vi "Start measurement.vi"(10 "Actual measurement":T2={"Start"=80.0, "Start Caption"="Start [T]", "End"=0.0, "End Caption"="End [T]", "Sweep"=0.0, "Sweep caption"="Rate [mT/s]", "Constant"=0.0, "Constant caption"="Freq [GHz]", "Mod_F [kHz]"=0.0, "Mod_A [G]"=0.001, "Tau [ms]"=0.0, "Angle [°]"=0.0, "Tmp [K]"=50.0, "Wait [min]"=0.0, "Carousel"=-1, "Comment"="", "Auto-mod"=TRUE, "Execute"=FALSE} {"Carousel" items=["0", "1", "2", "3", "4", "5", "6"]; "Angle [°]" min=0.0 max=350.0; "Tau [ms]" min=0.0 max=100.0; "Wait [min]" min=0.0 max=350.0; "Tmp [K]" min=0.0 max=3000.0; "Mod_A [G]" min=0.1 max=150.0; "Mod_F [kHz]" min=0.1 max=150.0}, 11 "Referencies in":T1) -> (0 "error out":errorcluster)   [LabVIEW 2024]
uses:
  Datatypes/script polymorh line.ctl
  Subsystem modules/Messenger service/Data types/Messenger referencies.ctl
  Subsystem modules/Magnet module/ctl/SetField data.ctl
  Subsystem modules/Magnet module/ctl/Magnet mode public.ctl
  Subsystem modules/Magnet module/ctl/MSG to magnet.ctl
  Subsystem modules/Magnet module/ctl/Magnet Orders.ctl
  Subsystem modules/Lock-in module/ctl/MFLI_parameter and value.ctl
  Subsystem modules/Lock-in module/ctl/MFLI_node.ctl
  Subsystem modules/Lock-in module/ctl/MFLI_message for module.ctl
  Subsystem modules/Lock-in module/ctl/MFLI_command enum.ctl
  Subsystem modules/Sample rotator/ctl/MSG to Rotator.ctl
  Subsystem modules/Sample rotator/ctl/Rotator commands.ctl
  Subsystem modules/Magnet module/Magnet module.lvlib
  Subsystem modules/Lock-in module/Lock-in module.lvlib
  Subsystem modules/Sample rotator/SampleRotator.lvlib
  Subsystem modules/Messenger service/MessengerLib.lvlib
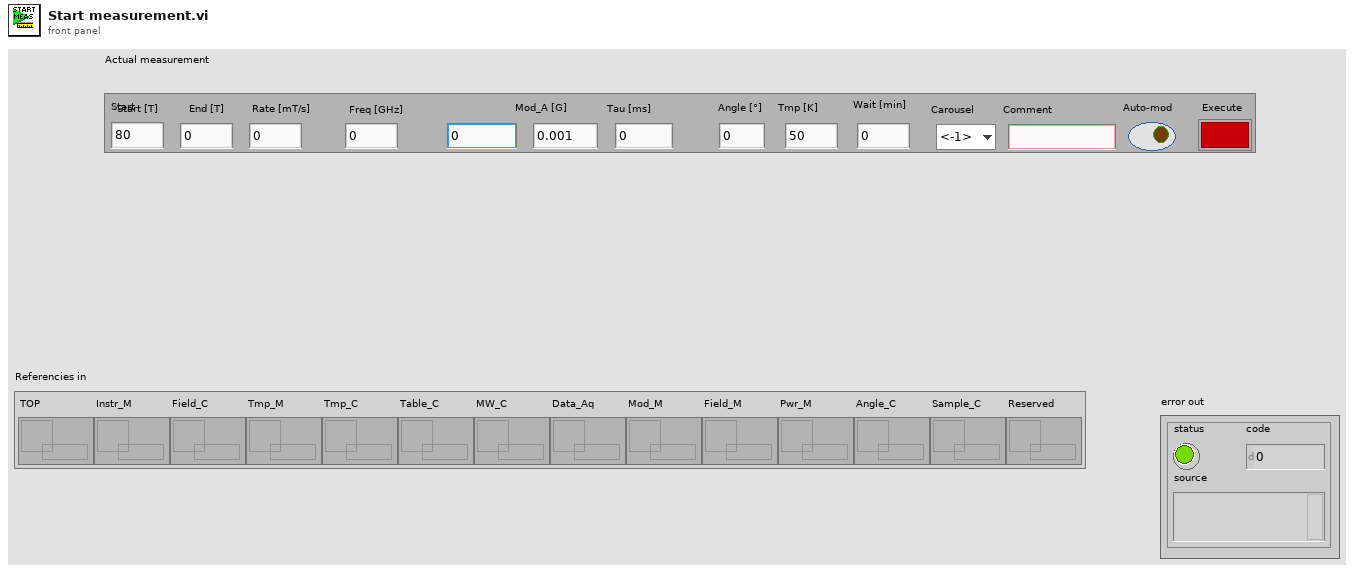
[diagram p1: front panel]
types:
  T1 = typedef "MessengerLib.lvlib/Messenger referencies.ctl" = cluster{"TOP":refnum<queue>, "Instr_M":refnum<queue>, "Field_C":refnum<queue>, "Tmp_M":refnum<queue>, "Tmp_C":refnum<queue>, "Table_C":refnum<queue>, "MW_C":refnum<queue>, "Data_Aq":refnum<queue>, "Mod_M":refnum<queue>, "Field_M":refnum<queue>, "Pwr_M":refnum<queue>, "Angle_C":refnum<queue>, "Sample_C":refnum<queue>, "Reserved":refnum<queue>}
  T2 = typedef "script polymorh line.ctl" = cluster{"Start":dbl, "Start Caption":string, "End":dbl, "End Caption":string, "Sweep":dbl, "Sweep caption":string, "Constant":dbl, "Constant caption":string, "Mod_F [kHz]":dbl, "Mod_A [G]":dbl, "Tau [ms]":dbl, "Angle [°]":dbl, "Tmp [K]":dbl, "Wait [min]":dbl, "Carousel":i8, "Comment":string, "Auto-mod":bool, "Execute":bool}
  T3 = typedef "Magnet module.lvlib/MSG to magnet.ctl" = cluster{"Order":T4, "Data":variant}
  T4 = typedef "Magnet module.lvlib/Magnet Orders.ctl" = enum16{"Ignore", "Connect", "Update", "Switch mode", "Set field", "Stop ramping", "Equalize output", "Zero output", "Flip polarity", "Blackout", "Set timer", "Eval temperatures", "Disconnect"}
  T5 = typedef "Lock-in module.lvlib/MFLI_message for module.ctl" = cluster{"Command":T6, "Data":variant}
  T6 = typedef "Lock-in module.lvlib/MFLI_command enum.ctl" = enum16{"Initialize", "Update", "Set parameters", "Set module", "Set individual parameters", "Get point", "Get array", "Disconnect", "End", "Ignore"}
  T7 = typedef "Lock-in module.lvlib/MFLI_parameter and value.ctl" = cluster{"parameter":T8, "value":dbl}
  T8 = typedef "Lock-in module.lvlib/MFLI_node.ctl" = enum16{"None", "filter_order [-]", "filter_constant [ms]", "in_diff", "in_autorange", "in_imp50", "in_AC", "osc_freq [kHz]", "out_ampl [V]", "out_autorange", "out_imp50", "enable output", "enamble ampl", "scope_enable", "scope_rate", "scope_len", "scope_trigEn", "AuxOut_amplify", "Phase_deg", "AuxOut_select"}
  T9 = typedef "Magnet module.lvlib/Magnet mode public.ctl" = enum16{"Persistant", "Ramping"}
  T10 = typedef "Magnet module.lvlib/SetField data.ctl" = cluster{"Field [T]":dbl, "Ramp [T/s]":dbl, "Custom Ramp?":bool, "Mode":T9}
  T11 = typedef "SampleRotator.lvlib/MSG to Rotator.ctl" = cluster{"Command":T12, "Data":variant}
  T12 = typedef "SampleRotator.lvlib/Rotator commands.ctl" = enum16{"Ignore", "Initialize", "Update", "Set parameters", "Stop movement", "Set position", "Disconnect", "End"}
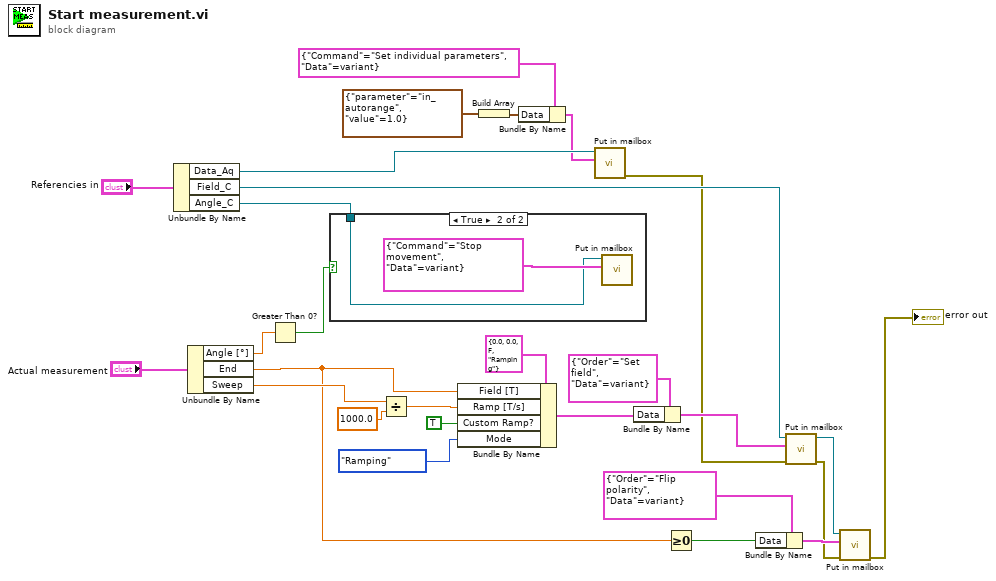
[diagram p0: block diagram]
diagram:
  n1 = Unbundle By Name("Referencies in") -> ("Data_Aq"=w14:refnum<queue>, "Field_C"=w7:refnum<queue>, "Angle_C"=w2:refnum<queue>)
  n2 = Unbundle By Name("Actual measurement") -> ("Angle [°]"=w3:dbl, "End"=w26:dbl, "Sweep"=w27:dbl)
  n3 = Greater Than 0?(x=w3) -> (x > 0?=w1:bool)
  n4 = case shown="True" w1 {
    tunnel: w2 -> [_ w29]
    frame False {
    }
    frame True {
      n5 = call "Put in mailbox.vi"("Message"=T11 {"Command"=enum."Stop movement", "Data"=variant} ("MSG to rotator"), "Queue in"=w29) -> ()  [unwired: 7 in, 3 out]
    }
  }
  n6 = Divide(x=w27, y=1000.0) -> (x/y=w23:dbl)
  n7 = Bundle By Name(cluster=T10 {"Field [T]"=0.0, "Ramp [T/s]"=0.0, "Custom Ramp?"=FALSE, "Mode"=enum."Ramping"} ("Set Field"), "Field [T]"=w26, "Ramp [T/s]"=w23, "Custom Ramp?"=TRUE, "Mode"=Magnet_mode_public."Ramping") -> (w22:T10)
  n8 = Build Array(T7 {"parameter"=enum."in_autorange", "value"=1.0} ("Parameter to set")) -> (w12:T7[])
  n9 = Bundle By Name(cluster=T5 {"Command"=enum."Set individual parameters", "Data"=variant} ("MSG for  ACQ"), "Data"=w12) -> (w11:T5)
  n10 = call "Put in mailbox.vi"("Message"=w11, "Queue in"=w14) -> ("error out"=w5:errorcluster)  [unwired: 7 in, 2 out]
  n11 = Bundle By Name(cluster=T3 {"Order"=enum."Set field", "Data"=variant} ("MSG to magnet"), "Data"=w22) -> (w21:T3)
  n12 = Greater Or Equal To 0?(x=w26) -> (x >= 0?=w8:bool)
  n13 = Bundle By Name(cluster=T3 {"Order"=enum."Flip polarity", "Data"=variant} ("MSG to magnet"), "Data"=w8) -> (w9:T3)
  n14 = call "Put in mailbox.vi"("error in (no error)"=w5, "Message"=w21, "Queue in"=w7) -> ("error out"=w4:errorcluster, "Queue out"=w6:refnum<queue>)  [unwired: 6 in, 1 out]
  n15 = call "Put in mailbox.vi"("error in (no error)"=w4, "Message"=w9, "Queue in"=w6) -> ("error out"=→"error out":errorcluster)  [unwired: 6 in, 2 out]
